vi "Apply DevInfo.vi"(8 "error in (no error)":errorcluster, 10 "DevInfo":refnum<class "DevInfo.lvclass">, 11 "CCD in":refnum<class "CCD.lvclass">) -> (0 "error out":errorcluster, 3 "CCD out":refnum<class "CCD.lvclass">)   [LabVIEW 2016, in "CCD.lvlib" / "CCD.lvclass"]
uses:
  <userlib>/Common Components/Hardware/CCD/CCD/CCD.lvclass
  <userlib>/Common Components/Hardware/DevInfo/DevInfo.lvclass
  <userlib>/Common Components/Hardware/Abstract Hardware/Hardware.lvclass
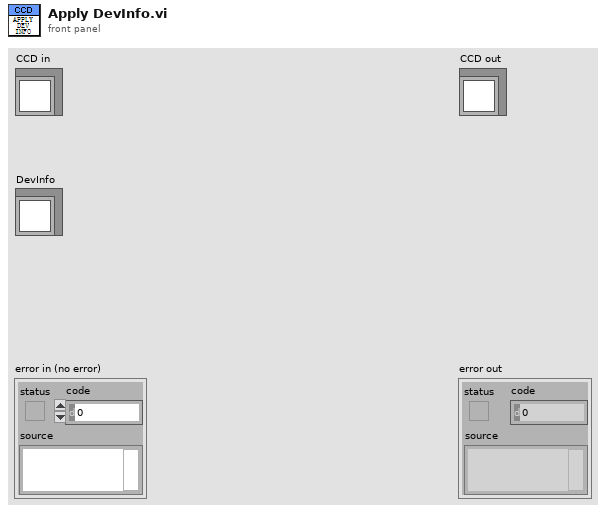
[diagram p1: front panel]
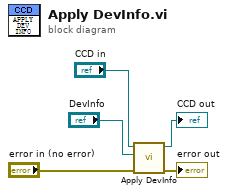
[diagram p0: block diagram]
diagram:
  n1 = call-parent "Apply DevInfo.vi"("error in (no error)"="error in (no error)", "DevInfo"="DevInfo", "Hardware in"="CCD in") -> ("error out"=→"error out":errorcluster, "Hardware out"=→"CCD out":refnum<class "CCD.lvclass">)  [unwired: 7 in]
